vi "Modbus_Lee.vi"() -> (3 "register values":u16[](array[numeric]))   [LabVIEW 2019, in "Class 2.lvclass"]
uses:
  Class 2.lvclass
  <vilib>/NI/Modbus Library/API/Wrapper/Create TCP Master.vi
  <vilib>/NI/Modbus Library/API/Master/Modbus Master.lvclass
  <vilib>/NI/Modbus Library/API/Wrapper/API Main.lvlib
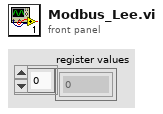
[diagram p1: front panel]
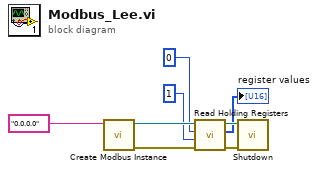
[diagram p0: block diagram]
diagram:
  n1 = call-poly <vilib>:"Create Modbus Instance.vi"("address"="0.0.0.0") -> ("error out"=w6:errorcluster, "TCP master instance"=w7:refnum<class "Modbus Master.lvclass">)  [unwired: 9 in]
  n2 = call-dynamic "Read Holding Registers.vi"("error in"=w6, "number of inputs"=u16 1, "starting address"=u16 0, "Modbus master in"=w7) -> ("error out"=w4:errorcluster, "register values"=→"register values":u16[], "Modbus master out"=w5:refnum<class "Modbus Master.lvclass">)  [unwired: 5 in]
  n3 = call-dynamic "Shutdown.vi"("error in"=w4, "Modbus master in"=w5) -> ()  [unwired: 9 in, 1 out]
